vi "writeU16FIFO.vi"(8 "error in (no error)":errorcluster, 9 "Timeout":i32, 10 "Data":u16[](array[numeric]), 11 "IWriteU16FIFO in":refnum<class "IWriteU16FIFO.lvclass">) -> (0 "error out":errorcluster, 2 "ElementsRemaining":u32, 3 "IWriteU16FIFO out":refnum<class "IWriteU16FIFO.lvclass">)   [LabVIEW 2015, in "RTFPGA.lvlib" / "IWriteU16FIFO.lvclass"]
uses:
  IWriteU16FIFO.lvclass
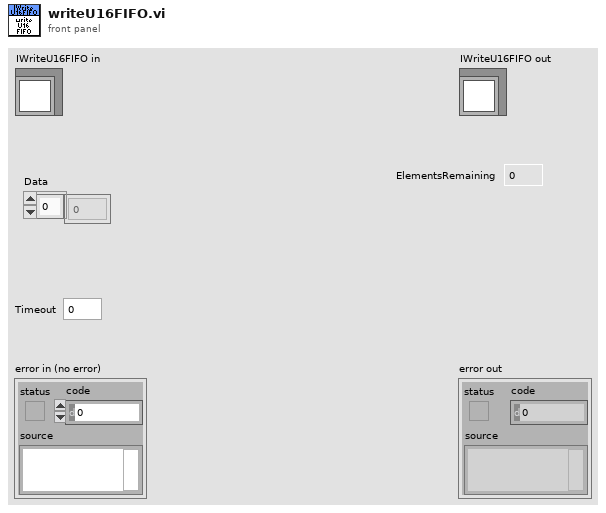
[diagram p1: front panel]
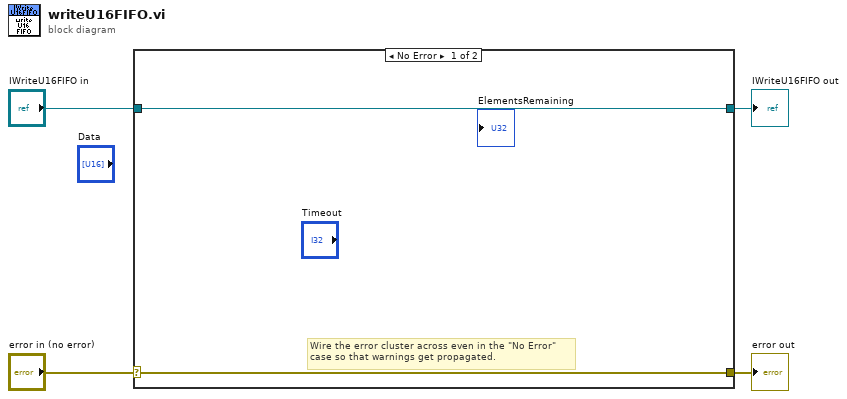
[diagram p0: block diagram]
diagram:
  n1 = case shown="No Error" "error in (no error)" {
    selector: "error in (no error)" -> [w5 w8]
    tunnel: [w5 w8] -> w3
    tunnel: [w6 w7] -> w1
    tunnel: "IWriteU16FIFO in" -> [w6 w7]
    frame No Error {
      # "Wire the error cluster across even in the \"No Error\"\ncase so that warnings get propagated."
    }
    frame Error {
    }
  }
  "error out" <- w3
  "IWriteU16FIFO out" <- w1
